vi "Position Cancel Button.vi"(8 "error in (no error)":errorcluster, 10 "Title String":refnum<vi>, 11 "Cancel Button":refnum<vi>) -> (0 "error out":errorcluster)   [LabVIEW 2014]
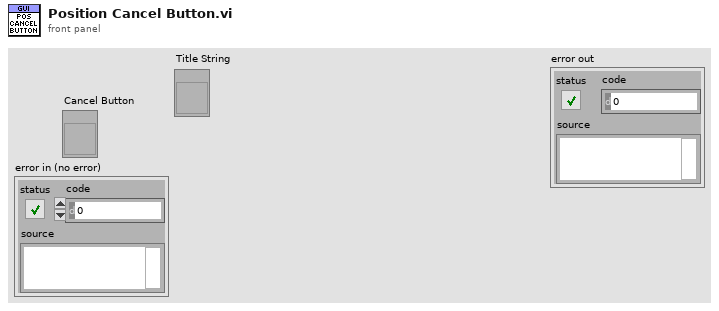
[diagram p1: front panel]
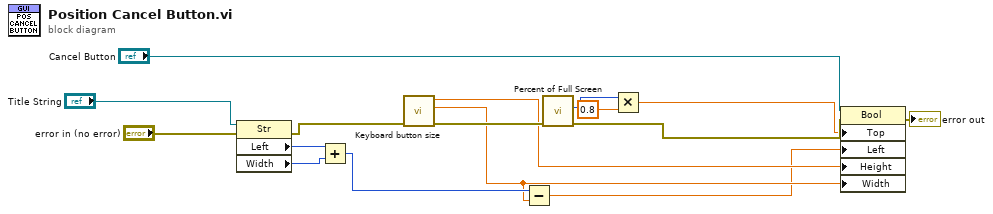
[diagram p0: block diagram]
diagram:
  n1 = property class="Str"(reference="Title String", error in="error in (no error)") -> (error out=w11:errorcluster, "Left"=w5:i32, "Width"=w4:u32)  [unwired: 1 out]
  n2 = Add(x=w5, y=w4) -> (x+y=w3:u32)
  n3 = call "Keyboard button size.vi"("error in (no error)"=w11) -> ("error out"=w10:errorcluster, "Key Width"=w2:dbl, "Key Height"=w6:dbl)  [unwired: 7 in, 1 out]
  n4 = Subtract(x=w3, y=w2) -> (x-y=w1:dbl)
  n5 = call "Percent of Full Screen.vi"("error in (no error)"=w10) -> ("error out"=w16:errorcluster, "Bottom"=w9:i16)  [unwired: 8 in, 1 out]
  n6 = Multiply(x=w9, y=0.8) -> (x*y=w7:dbl)
  n7 = property class="Bool"(reference="Cancel Button", error in=w16, "Top"=w7, "Left"=w1, "Height"=w6, "Width"=w2) -> (error out=→"error out":errorcluster)  [unwired: 1 out]
